vi "__uintAdd.vi"(3 "Base (decimal)":T2=10 items=["Binary"=2, "Octal"=8, "Decimal"=10, "Hexadecimal"=16, "Hexatrigesimal"=36, "ASCII"=64], 4 "Timeout (-1)":T1=-1, 5 "Uint2 in":u8[](array[numeric])=[0], 6 "Uint1 in":u8[](array[numeric])=[0]) -> (0 "Timing":u32, 1 "Timeout?":bool, 2 "Uint1 + Uint2":u8[](array[numeric]))   [LabVIEW 2011, in "UintClass.lvclass"]
uses:
  UintClass.lvclass
  enumBase.ctl
  timeout.ctl
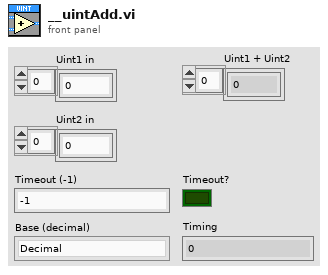
[diagram p1: front panel]
types:
  T1 = typedef "UintClass.lvclass/timeout.ctl" = i32
  T2 = typedef "UintClass.lvclass/enumBase.ctl" = u16
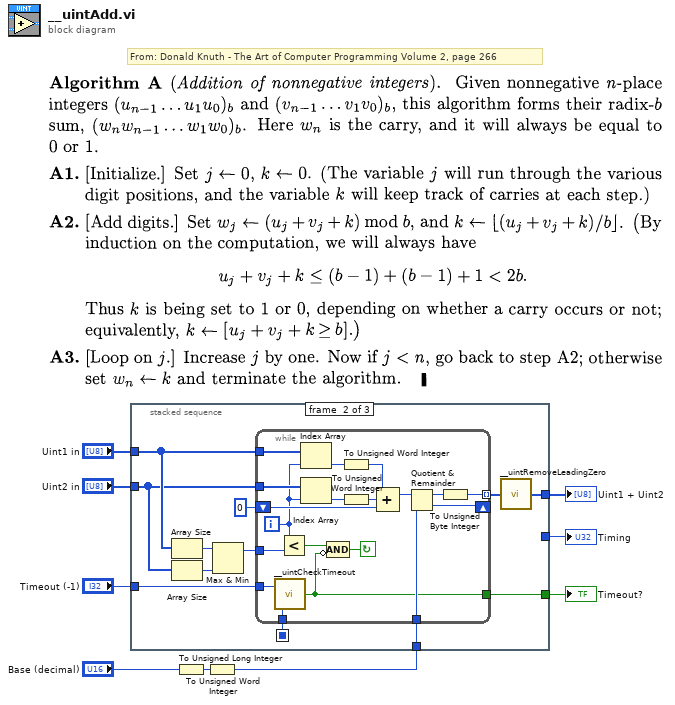
[diagram p0: block diagram]
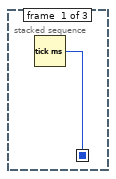
[diagram p2: hidden frame]
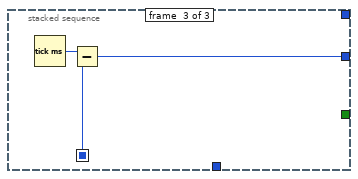
[diagram p3: hidden frame]
diagram:
  # "From: Donald Knuth - The Art of Computer Programming Volume 2, page 266"
  n1 = To Unsigned Long Integer(number="Base (decimal)") -> (unsigned 32bit integer=w6:u32)
  n2 = To Unsigned Word Integer(number=w6) -> (unsigned 16bit integer=w5:u16)
  n3 = stacked-sequence {
    seq-local: [w10 _ _] -> [_ w12 w43]
    tunnel: "Uint1 in" -> [_ w20 _]
    tunnel: "Uint2 in" -> [_ w19 _]
    tunnel: [_ w17 _] -> w9
    tunnel: w5 -> [_ w15 _]
    tunnel: [_ _ w42] -> w3
    tunnel: "Timeout (-1)" -> [_ w13 _]
    tunnel: [_ w11 _] -> w1
    frame #0 {
      n4 = Tick Count (ms)() -> (millisecond timer value=w10:u32)
    }
    frame #1 {
      n5 = Array Size(array=w20) -> (size(s)=w22:i32)
      n6 = Array Size(array=w19) -> (size(s)=w21:i32)
      n7 = Max & Min(x=w22, y=w21) -> (max(x,y)=w14:i32)  [unwired: 1 out]
      n8 = while {
        tunnel: w20 -> [w41]
        tunnel: w19 -> [w40]
        shift-right: [w29] -> _
        shift-left: u16 0 -> [w37]
        tunnel: w14 -> [w35]
        tunnel: [w33] -> w18 mode=indexing
        tunnel: w15 -> [w28]
        tunnel: w13 -> [w27]
        tunnel: w12 -> [w26]
        tunnel: [w23] -> w11
        i -> [w36]
        stop <- w25 continue-if-true
        n9 = call "__uintCheckTimeout.vi"("Millisecond timer value"=w26, "Timeout (-1)"=w27) -> ("Timeout?"=w23:bool)
        n10 = Less?(x=w36, y=w35) -> (x < y?=w24:bool)
        n11 = Index Array(array=w41, index=w36) -> (element=w39:u8)
        n12 = Index Array(array=w40, index=w36) -> (element=w38:u8)
        n13 = Compound Arithmetic op=AND(w24, invert w23) -> (w25:bool)
        n14 = To Unsigned Word Integer(number=w39) -> (unsigned 16bit integer=w32:u16)
        n15 = To Unsigned Word Integer(number=w38) -> (unsigned 16bit integer=w31:u16)
        n16 = Compound Arithmetic op=ADD(w32, w31, w37) -> (w30:u16)
        n17 = Quotient & Remainder(x=w30, y=w28) -> (x-y*floor(x/y)=w34:u16, floor(x/y)=w29:u16)
        n18 = To Unsigned Byte Integer(number=w34) -> (unsigned 8bit integer=w33:u8)
      }
      n19 = call "__uintRemoveLeadingZero.vi"("Uint in"=w18) -> ("Uint out"=w17:u8[])
    }
    frame #2 {
      n20 = Tick Count (ms)() -> (millisecond timer value=w44:u32)
      n21 = Subtract(x=w44, y=w43) -> (x-y=w42:u32)
    }
  }
  "Timing" <- w3
  "Uint1 + Uint2" <- w9
  "Timeout?" <- w1
